vi "check speedline file status.vi"(11 "makeSpeedlinesData in":T1) -> (3 "makeSpeedlinesData out":T1)   [LabVIEW 2018]
uses:
  make speedlines UI data.ctl
types:
  T1 = typedef "make speedlines UI data.ctl" = cluster{"folder":path, "PR Channel":u16, "Massflow Channel":u16, "speedlineCount":u16, "massFlowData":dbl[], "PRdata":dbl[], "progress":refnum<vi>, "PR":refnum<vi>, "massflow":refnum<vi>, "speedlineFileRef":refnum<file>, "speedlineFile":path, "speedlines":cluster{"mDot":dbl[], "PR":dbl[]}[]}
  T2 = enum16{"open", "replace", "create", "open or create", "replace or create", "replace or create with confirmation"}
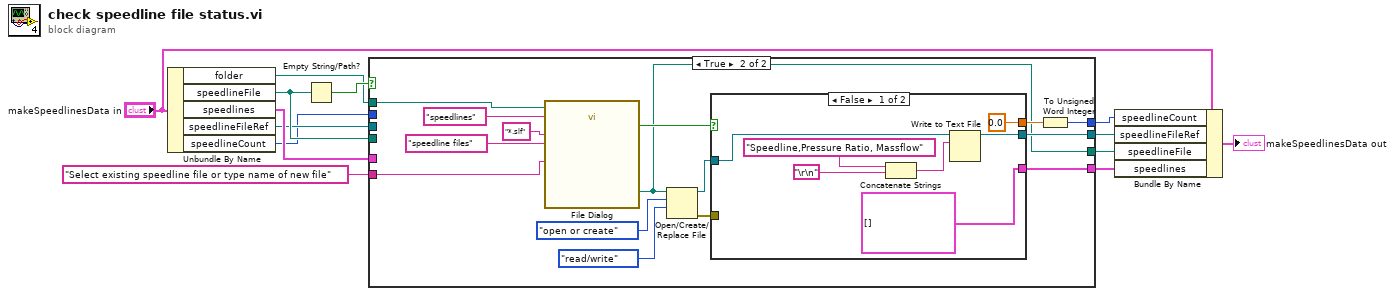
[diagram p0: block diagram]
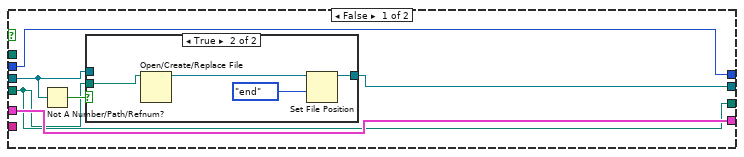
[diagram p2: hidden frame]
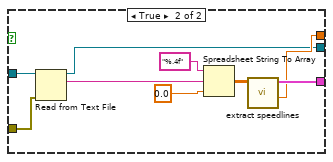
[diagram p4: hidden frame]
diagram:
  n1 = Unbundle By Name("makeSpeedlinesData in") -> ("folder"=w10:path, "speedlineFile"=w3:path, "speedlines"=w4:cluster{"mDot":dbl[], "PR":dbl[]}[], "speedlineFileRef"=w2:refnum<file>, "speedlineCount"=w1:u16)
  n2 = Empty String/Path?(string/path=w3) -> (empty?=w11:bool)
  n3 = case shown="True" w11 {
    tunnel: w10 -> [_ w39]
    tunnel: "Select existing speedline file or type name of new file" ("prompt") -> [_ w35]
    tunnel: [w19 w29] -> w8
    tunnel: [w14 w25] -> w7
    tunnel: [w16 w27] -> w6
    tunnel: [w17 w26] -> w5
    tunnel: w4 -> [w19 _]
    tunnel: w3 -> [w17 _]
    tunnel: w2 -> [w15 _]
    tunnel: w1 -> [w14 _]
    frame False {
      n4 = Not A Number/Path/Refnum?(number/path/refnum=w15) -> (NaN/Path/Refnum?=w18:bool)
      n5 = case shown="True" w18 {
        tunnel: w17 -> [_ w24]
        tunnel: [w20 w21] -> w16
        tunnel: w15 -> [w20 _]
        frame False {
        }
        frame True {
          n6 = Open/Create/Replace File(file path (use dialog)=w24) -> (refnum out=w23:refnum<file>)  [unwired: 5 in, 2 out]
          n7 = Set File Position(refnum=w23, from (0:start)=enum16{"start", "end", "current"}."end") -> (refnum out=w21:refnum<file>)  [unwired: 2 in, 1 out]
        }
      }
    }
    frame True {
      n8 = call "File Dialog"("start path"=w39, "prompt"=w35, "default name"="speedlines", "pattern (all files)"="*.slf", "pattern label"="speedline files") -> ("selected path"=w26:path, "exists"=w32:bool)  [unwired: 7 in, 2 out]
      n9 = Open/Create/Replace File(file path (use dialog)=w26, operation (0:open)=T2."open or create", access (0:read/write)=enum16{"read/write", "read-only", "write-only"}."read/write") -> (refnum out=w31:refnum<file>, error out=w30:errorcluster)  [unwired: 3 in, 1 out]
      n10 = case shown="False" w32 {
        tunnel: w31 -> [w46 w55]
        tunnel: w30 -> [_ w54]
        tunnel: [cluster{dbl[], dbl[]}[] [] ("speedlines") w49] -> w29
        tunnel: [0.0 ("speedlineID") w48] -> w28
        tunnel: [w45 w47] -> w27
        frame False {
          n11 = Concatenate Strings("Speedline,Pressure Ratio, Massflow" ("text"), "\r\n") -> (w40:string)
          n12 = Write to Text File(file (use dialog)=w46, text=w40) -> (refnum out=w45:refnum<file>)  [unwired: 2 in, 2 out]
        }
        frame True {
          n13 = Read from Text File(file (use dialog)=w55, error in=w54) -> (refnum out=w47:refnum<file>, text=w53:string)  [unwired: 2 in, 2 out]
          n14 = Spreadsheet String To Array(format string="%.4f", spreadsheet string=w53, array type (2D Dbl)=0.0) -> (array=w50:dbl[][])  [unwired: 1 in]
          n15 = call "extract speedlines.vi"("speedlineFileData"=w50) -> ("speedlineID"=w48:dbl, "speedlines"=w49:cluster{dbl[], dbl[]}[])  [unwired: 9 in]
        }
      }
      n16 = To Unsigned Word Integer(number=w28) -> (unsigned 16bit integer=w25:u16)
    }
  }
  n17 = Bundle By Name(cluster="makeSpeedlinesData in", "speedlineCount"=w7, "speedlineFileRef"=w6, "speedlineFile"=w5, "speedlines"=w8) -> (→"makeSpeedlinesData out":T1)
